vi "getTestsFromTestCaseObject.vi"(8 "error in":errorcluster, 11 "Test in":refnum<class>) -> (0 "error out":errorcluster, 2 "Test Method Names":string[](array[string]), 3 "Test out":refnum<class>)   [LabVIEW 2013, in "TestLoader.lvclass"]
uses:
  TestLoader.lvclass
  Libraries/VITesterUtilities.lvlib
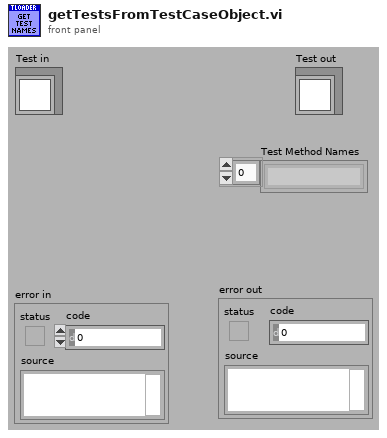
[diagram p1: front panel]
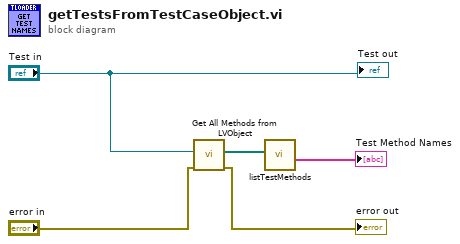
[diagram p0: block diagram]
diagram:
  n1 = call "Get All Methods from LVObject.vi"("error in"="error in", "LabVIEW Object"="Test in") -> ("error out"=→"error out":errorcluster, "Methods"=w2:path[])  [unwired: 8 in]
  n2 = call "listTestMethods.vi"("Methods"=w2) -> ("Test Method Names"=→"Test Method Names":string[])  [unwired: 9 in, 1 out]
  "Test out" <- "Test in"
